vi "Script_Generator.vi"() -> ()   [LabVIEW 2013]
uses:
  Global_Not-Aus.vi
  <vilib>/Utility/file.llb/Read From Spreadsheet File (string).vi
  <vilib>/Utility/file.llb/Write To Spreadsheet File (string).vi
panel:
  out "Abs_pos":string[](array[string])
  out "Array - String":string[][](array[string])
  in  "Main Tab":enum32{"Page 1"}(tab)
  out "Generated Sequence":string[][](array[string])
  in  "Set/Write/Read":enum32{"Position Set", "Write", "Read"}(tab)
  in  "Position Set":T1(tab)
  in  "Generate P1":bool
  in  "Speed (P)":dbl min=0.0 max=20.0
  in  "Generate P2":bool
  in  "Position":T2(ring)
  in  "Proceed W/R":bool
  in  "Generate P3":bool
  in  "Z(P)":string(combo)
  in  "Y(P)":string(combo)
  in  "X(P)":string(combo)
  in  "Z axis":dbl
  in  "Y axis":dbl
  in  "X axis":dbl
  in  "Write_Menu":T3(tab)
  in  "Generate W1":bool
  in  "Speed (W)":dbl min=0.0 max=20.0
  in  "Proceed Inc/Abs":bool
  in  "Current":dbl min=0.0 max=10.0 step=0.1
  in  "Generate W2":bool
  in  "Incre/abs":enum32{"Incremental", "Absolute"}(tab)
  in  "Z_axis(Inc)":string(combo)
  in  "Y_axis(Inc)":string(combo)
  in  "X_axis(Inc)":string(combo)
  in  "Z_axis":dbl
  in  "Y_axis":dbl
  in  "X_axis":dbl
  in  "Incremental":bool
  in  "Strip Length":dbl
  in  "Pole width N":dbl min=0.0 max=10.0 step=0.1
  in  "Pole width S":dbl min=0.0 max=10.0 step=0.1
  in  "Start Pole (N/S)":string(combo)
  in  "Z_axis(Abs)":string(combo)
  in  "Y_axis(Abs)":string(combo)
  in  "X_axis(Abs)":string(combo)
  in  "Start_Pole(N/S)":string(combo)
  in  "Absolute":bool
  in  "Select File":path=path "Y:/01_Projekte/EPN93031_Schreibplatz/8_Konstruktionsunterlagen/8.5_Software/COPY_KOSY Steuerung LabVIEW/1.New_Code_2014_2015/noniuos_scale.txt"
  in  "Generate W4":bool
  in  "File Path_Write":path=path "Y:/01_Projekte/EPN93031_Schreibplatz/8_Konstruktionsunterlagen/8.5_Software/COPY_KOSY Steuerung LabVIEW/1.New_Code_2014_2015/New_Scripts/sample_write.txt"
  in  "Read_Menu":T4(tab)
  in  "Generate R1":bool
  in  "Z(R)":string(combo)
  in  "Y(R)":string(combo)
  in  "X(R)":string(combo)
  in  "Zaxis":dbl min=0.0 max=10.0 step=0.1 format="%#_6f"
  in  "Yaxis":dbl min=0.0 max=10.0 step=0.1 format="%#_2f"
  in  "Xaxis":dbl min=0.0 max=10.0 step=0.1 format="%#_6f"
  out "Count":dbl
  in  "Strip_Length":dbl
  in  "Move&Measure":bool
  in  "Continuous":bool
  in  "Generate R2":bool
  in  "ED32i":bool
  in  "ED33":bool
  in  "KMT":bool
  in  "Generate R4":bool
  in  "File Path_Read":path=path "Y:/01_Projekte/EPN93031_Schreibplatz/8_Konstruktionsunterlagen/8.5_Software/COPY_KOSY Steuerung LabVIEW/1.New_Code_2014_2015/New_Scripts/sample_read.txt"
  in  "Clear Sequence":bool
  in  "Stop Program":bool
  # "SCRIPT GENERATOR  V1.0"
  # "Position Set\n\n1. Speed - Set the speed for the movement to initial \n                   position and press 'OK'.\n2. Batch Position - Select the 'Position' from the dropdown \n                   and press 'OK'.\n3. Movement - Select the number of steps(in mm) for \n                    movement in corresponding axis and also \n                    the direction of travel in the selected axis. \n                    Then press 'OK'."
  # "Speed - Set the speed for the writing process \n                and press 'OK'."
  # "Power - Set the 'Current' from the writing head \n                and press 'OK'."
  # "Incremental Writing Process\n \n1.Set the total 'length' of the strip.\n2.Set the 'Pole width N & S' to be magnetised.\n3.Select the N/S for the initial pole tab. \n3.Set the direction of travel in the selected axis.\n   Then press 'OK'."
  # "Absolute Writing\n\n1. Select the file from 'Select File' for nonious scale.\n2.Select the N/S for the initial pole tab. \n3.Set the direction of travel in the selected axis.\n   Then press 'OK'."
  # "Save Script - Select the file to which the generated \n                         script should be saved and the press 'OK'."
  # "Read\n\n1. Step & Count - 1. Set the total 'length' of the strip.\n                                 2. The 'Count' is automatically generated.\n                                 3. Set the number of steps(in mm) for \n                                     movement in corresponding axis and\n                                     also the direction of travel in the \n                                     selected axis. Then press 'OK'.\n2. Sensors -           Select the 'sensors' to be activated and \n                                 the type of measurement. Then press 'OK'.\n3. Save Script  -    Select the file to which the generated \n                                 script should be saved and the press 'OK'."
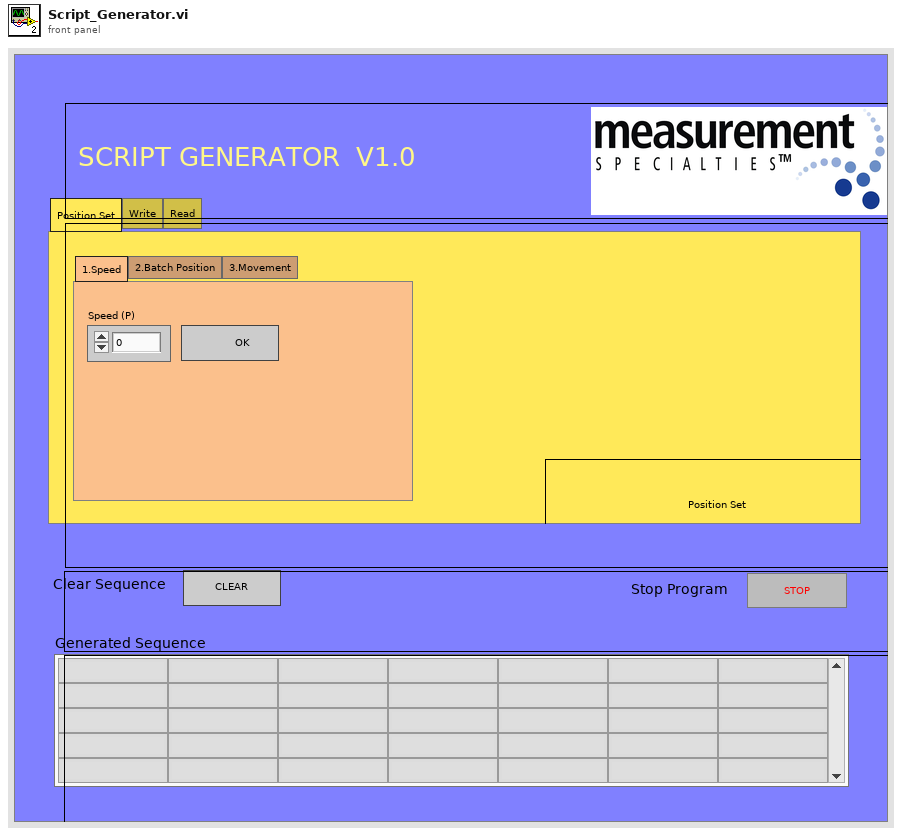
[diagram p1: front panel]
types:
  T1 = enum32{"1.Speed", "2.Batch Position", "3.Movement"}
  T2 = enum16{"Position 1", "Position 2", "Position 3", "Position 4", "Position 5", "Position 6", "Position 7", "Position 8", "Position 9", "Position 10"}
  T3 = enum32{"1.Speed", "2.Power", "3.Movement", "4.Save Script"}
  T4 = enum32{"1.Steps & Count", "2.Sensors", "3.Save Script"}
  T5 = enum16{"1.Speed", "2.Batch Position", "3.Movement"}
  T6 = enum32{"Page Enabled", "Page Disabled", "Page Disabled & Grayed"}
  T7 = enum16{"1.Steps & Count", "2.Sensors", "3.Save Script"}
  T8 = enum16{"1.Speed", "2.Power", "3.Movement", "4.Save Script"}
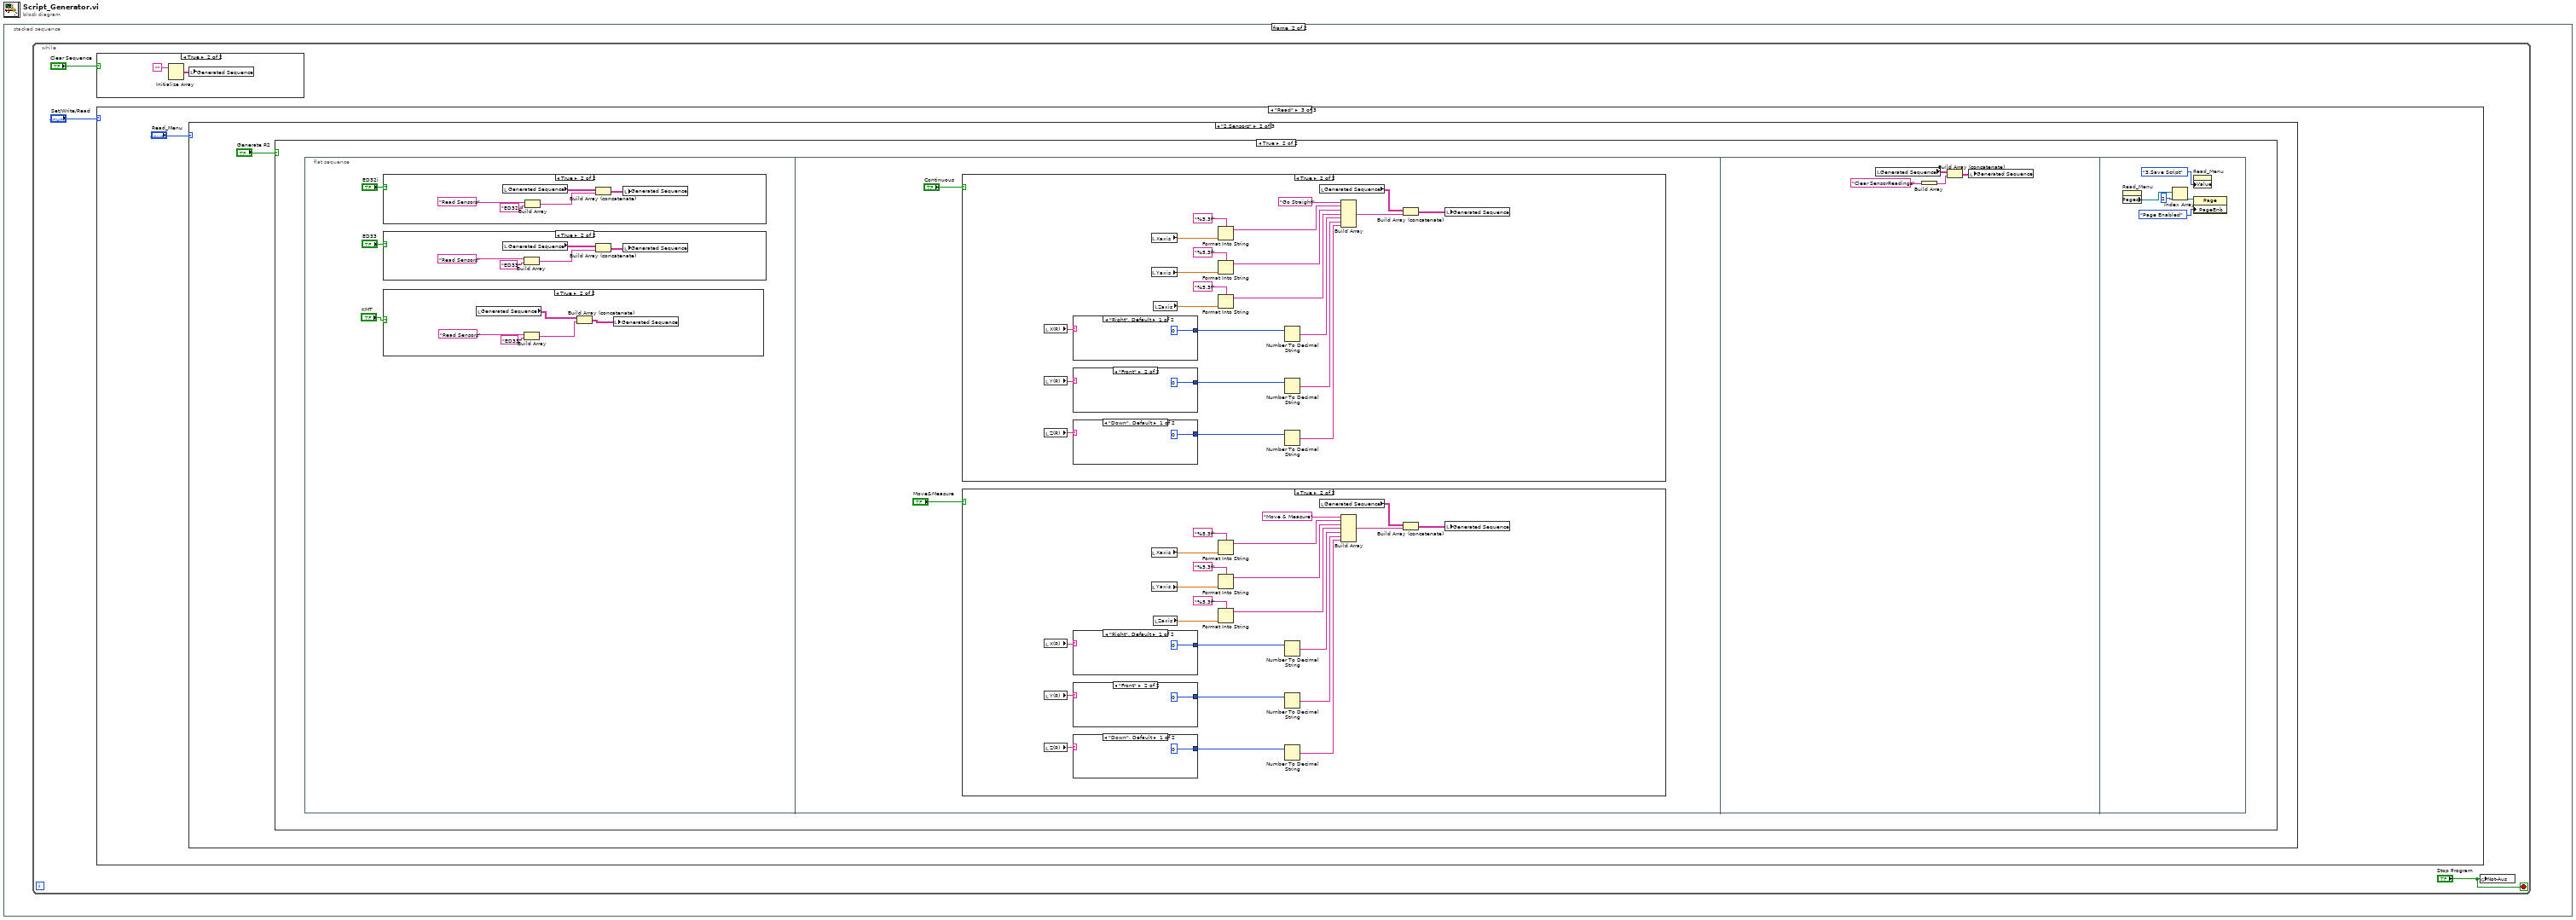
[diagram p0: block diagram]
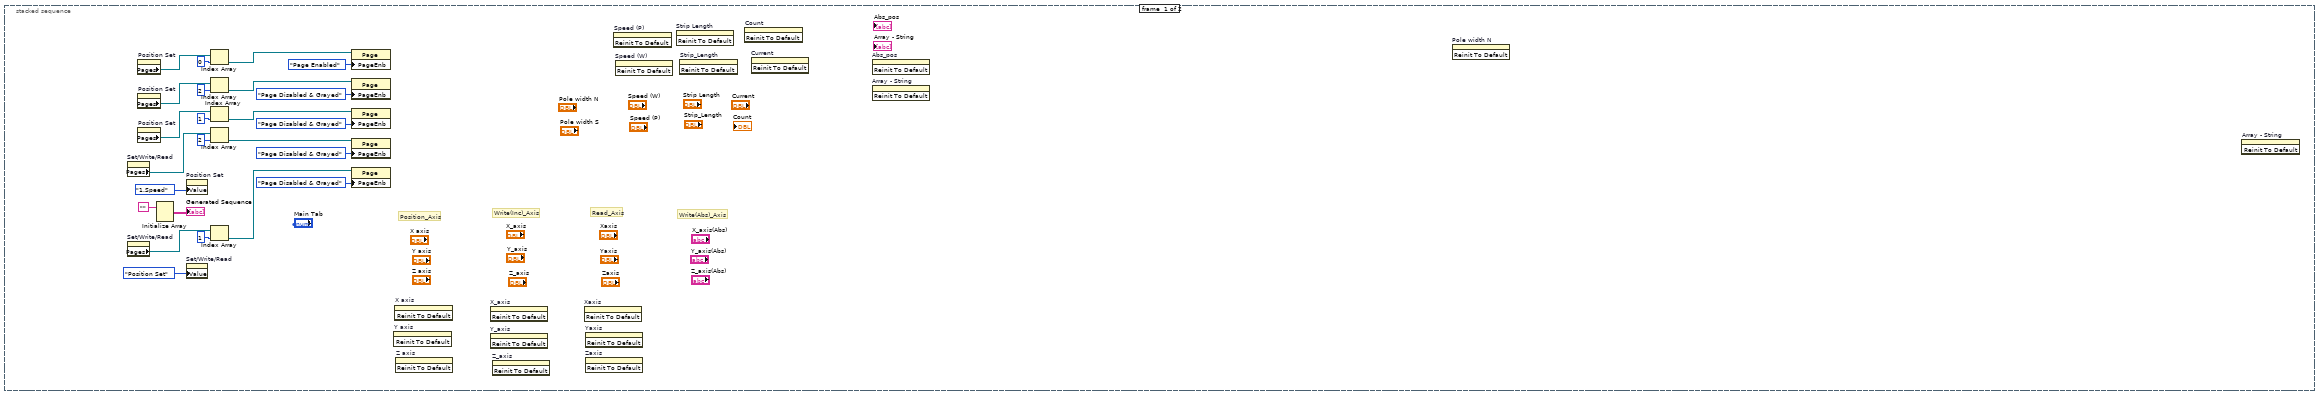
[diagram p2: hidden frame]
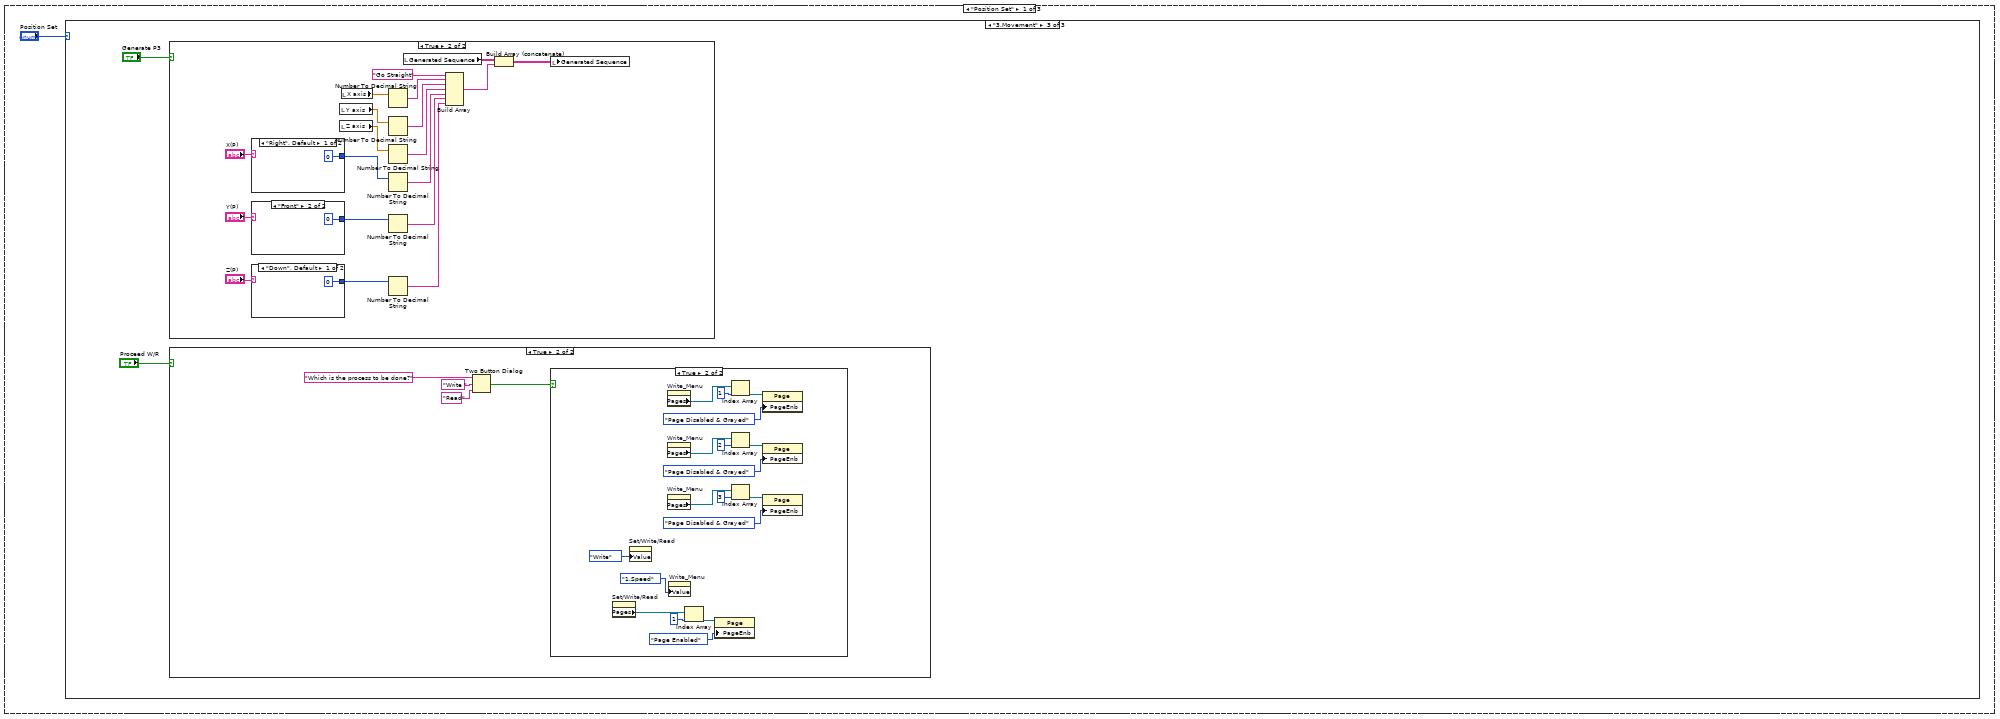
[diagram p4: hidden frame]
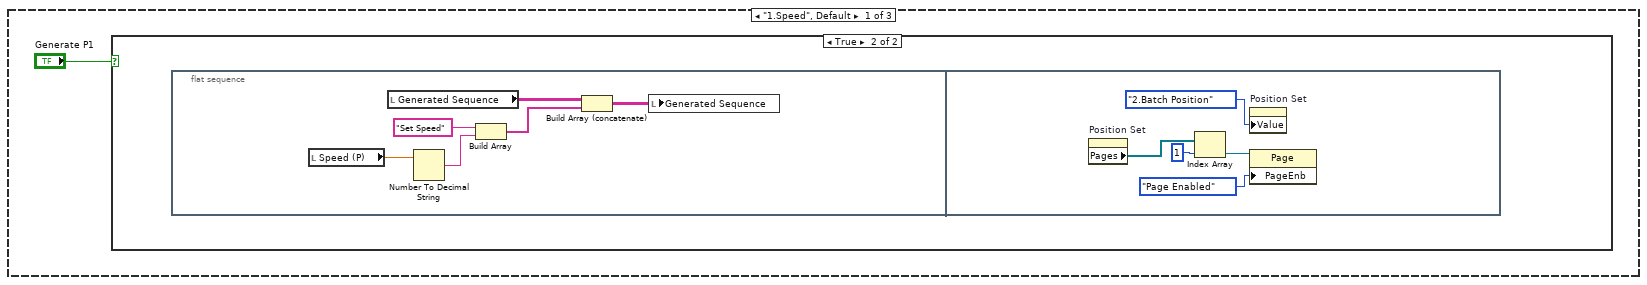
[diagram p5: hidden frame]
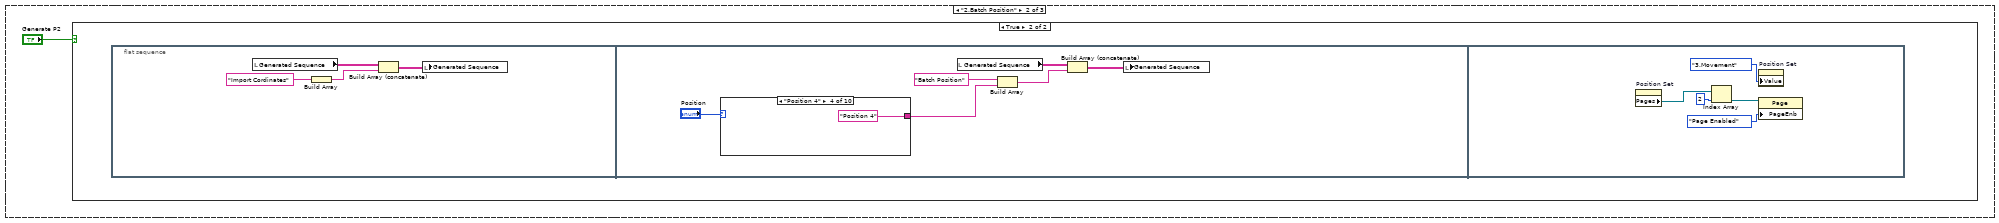
[diagram p7: hidden frame]
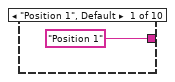
[diagram p9: hidden frame]
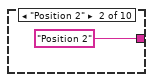
[diagram p10: hidden frame]
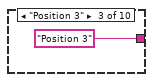
[diagram p11: hidden frame]
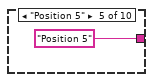
[diagram p12: hidden frame]
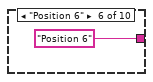
[diagram p13: hidden frame]
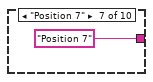
[diagram p14: hidden frame]
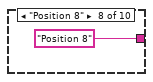
[diagram p15: hidden frame]
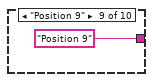
[diagram p16: hidden frame]
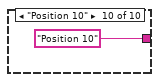
[diagram p17: hidden frame]
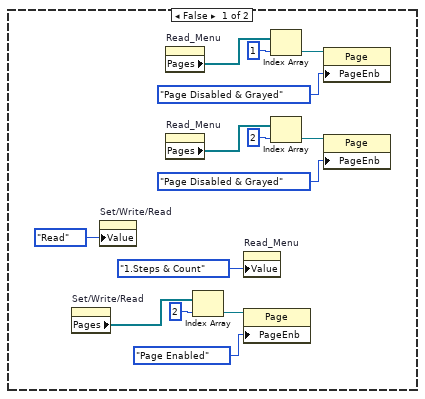
[diagram p19: hidden frame]
diagram:
  n1 = stacked-sequence {
    frame #0 {
      # "Write(Abs)_Axis"
      # "Read_Axis"
      # "Write(Inc)_Axis"
      # "Position_Axis"
      n2 = property on="Set/Write/Read" class="TabCtl (strict)"() -> ("Pages"=w16:refnum<vi>[])  [unwired: 2 in, 2 out]
      n3 = property on="Set/Write/Read" class="TabCtl (strict)"() -> ("Pages"=w15:refnum<vi>[])  [unwired: 2 in, 2 out]
      n4 = property on="Position Set" class="TabCtl (strict)"() -> ("Pages"=w14:refnum<vi>[])  [unwired: 2 in, 2 out]
      n5 = property on="Position Set" class="TabCtl (strict)"() -> ("Pages"=w13:refnum<vi>[])  [unwired: 2 in, 2 out]
      n6 = property on="Position Set" class="TabCtl (strict)"() -> ("Pages"=w3:refnum<vi>[])  [unwired: 2 in, 2 out]
      n7 = Initialize Array("") -> (→"Generated Sequence":string[][])  [unwired: 2 in]
      n8 = property on="Position Set" class="TabCtl (strict)"("Value"=T5."1.Speed") -> ()  [unwired: 2 in, 2 out]
      n9 = property on="Set/Write/Read" class="TabCtl (strict)"("Value"=enum16{"Position Set", "Write", "Read"}."Position Set") -> ()  [unwired: 2 in, 2 out]
      n10 = Index Array(array=w14, index=0) -> (element=w9:refnum<vi>)
      n11 = Index Array(array=w13, index=2) -> (element=w12:refnum<vi>)
      n12 = Index Array(array=w3, index=1) -> (element=w6:refnum<vi>)
      n13 = Index Array(array=w16, index=2) -> (element=w17:refnum<vi>)
      n14 = Index Array(array=w15, index=1) -> (element=w20:refnum<vi>)
      n15 = property class="Page"(reference=w9, "PageEnb"=T6."Page Enabled" ("Page Enabled State")) -> ()  [unwired: 1 in, 2 out]
      n16 = property class="Page"(reference=w12, "PageEnb"=T6."Page Disabled & Grayed" ("Page Enabled State")) -> ()  [unwired: 1 in, 2 out]
      n17 = property class="Page"(reference=w6, "PageEnb"=T6."Page Disabled & Grayed" ("Page Enabled State")) -> ()  [unwired: 1 in, 2 out]
      n18 = property class="Page"(reference=w17, "PageEnb"=T6."Page Disabled & Grayed" ("Page Enabled State")) -> ()  [unwired: 1 in, 2 out]
      n19 = property class="Page"(reference=w20, "PageEnb"=T6."Page Disabled & Grayed" ("Page Enabled State")) -> ()  [unwired: 1 in, 2 out]
      n20 = invoke on="Y axis" class="DigNum (strict)" method="Reinit To Default"() -> ()  [unwired: 3 in, 3 out]
      n21 = invoke on="X axis" class="DigNum (strict)" method="Reinit To Default"() -> ()  [unwired: 3 in, 3 out]
      n22 = invoke on="Z axis" class="DigNum (strict)" method="Reinit To Default"() -> ()  [unwired: 3 in, 3 out]
      n23 = invoke on="X_axis" class="DigNum (strict)" method="Reinit To Default"() -> ()  [unwired: 3 in, 3 out]
      n24 = invoke on="Y_axis" class="DigNum (strict)" method="Reinit To Default"() -> ()  [unwired: 3 in, 3 out]
      n25 = invoke on="Z_axis" class="DigNum (strict)" method="Reinit To Default"() -> ()  [unwired: 3 in, 3 out]
      n26 = invoke on="Xaxis" class="DigNum (strict)" method="Reinit To Default"() -> ()  [unwired: 3 in, 3 out]
      n27 = invoke on="Yaxis" class="DigNum (strict)" method="Reinit To Default"() -> ()  [unwired: 3 in, 3 out]
      n28 = invoke on="Zaxis" class="DigNum (strict)" method="Reinit To Default"() -> ()  [unwired: 3 in, 3 out]
      n29 = invoke on="Speed (P)" class="DigNum (strict)" method="Reinit To Default"() -> ()  [unwired: 3 in, 3 out]
      n30 = invoke on="Speed (W)" class="DigNum (strict)" method="Reinit To Default"() -> ()  [unwired: 3 in, 3 out]
      n31 = invoke on="Strip Length" class="DigNum (strict)" method="Reinit To Default"() -> ()  [unwired: 3 in, 3 out]
      n32 = invoke on="Strip_Length" class="DigNum (strict)" method="Reinit To Default"() -> ()  [unwired: 3 in, 3 out]
      n33 = invoke on="Count" class="DigNum (strict)" method="Reinit To Default"() -> ()  [unwired: 3 in, 3 out]
      n34 = invoke on="Current" class="DigNum (strict)" method="Reinit To Default"() -> ()  [unwired: 3 in, 3 out]
      n35 = invoke on="Abs_pos" class="Arr (strict)" method="Reinit To Default"() -> ()  [unwired: 3 in, 3 out]
      n36 = invoke on="Array - String" class="Arr (strict)" method="Reinit To Default"() -> ()  [unwired: 3 in, 3 out]
      n37 = invoke on="Pole width N" class="DigNum (strict)" method="Reinit To Default"() -> ()  [unwired: 3 in, 3 out]
      n38 = invoke on="Array - String" class="Arr (strict)" method="Reinit To Default"() -> ()  [unwired: 3 in, 3 out]
    }
    frame #1 {
      n39 = while {
        stop <- "Stop Program" stop-if-true
        n40 = case shown="True" "Clear Sequence" {
          frame False {
          }
          frame True {
            n41 = Initialize Array("") -> (w29:string[][])  [unwired: 2 in]
            n42 = local write "Generated Sequence"(w29) -> ()
          }
        }
        n43 = case shown="\"Read\"" "Set/Write/Read" {
          frame "Position Set" {
            n44 = case shown="\"3.Movement\"" "Position Set" {
              frame "1.Speed", Default {
                n45 = case shown="True" "Generate P1" {
                  frame False {
                  }
                  frame True {
                    n46 = flat-sequence {
                      frame #0 {
                        n47 = local read "Speed (P)"() -> (w37:dbl)
                        n48 = local read "Generated Sequence"() -> (w35:string[][])
                        n49 = Number To Decimal String(number=w37) -> (decimal integer string=w32:string)  [unwired: 1 in]
                        n50 = Build Array("Set Speed", w32) -> (w34:string[])
                        n51 = Build Array (concatenate)(w35, w34) -> (w36:string[][])
                        n52 = local write "Generated Sequence"(w36) -> ()
                      }
                      frame #1 {
                        n53 = property on="Position Set" class="TabCtl (strict)"() -> ("Pages"=w39:refnum<vi>[])  [unwired: 2 in, 2 out]
                        n54 = Index Array(array=w39, index=1) -> (element=w42:refnum<vi>)
                        n55 = property on="Position Set" class="TabCtl (strict)"("Value"=T5."2.Batch Position") -> ()  [unwired: 2 in, 2 out]
                        n56 = property class="Page"(reference=w42, "PageEnb"=T6."Page Enabled" ("Page Enabled State")) -> ()  [unwired: 1 in, 2 out]
                      }
                    }
                  }
                }
              }
              frame "2.Batch Position" {
                n57 = case shown="True" "Generate P2" {
                  frame False {
                  }
                  frame True {
                    n58 = flat-sequence {
                      frame #0 {
                        n59 = local read "Generated Sequence"() -> (w47:string[][])
                        n60 = Build Array("Import Cordinates") -> (w46:string[])
                        n61 = Build Array (concatenate)(w47, w46) -> (w44:string[][])
                        n62 = local write "Generated Sequence"(w44) -> ()
                      }
                      frame #1 {
                        n63 = case shown="\"Position 4\"" "Position" {
                          tunnel: ["Position 1" "Position 2" "Position 3" "Position 4" "Position 5" "Position 6" "Position 7" "Position 8" "Position 9" "Position 10"] -> w52
                          frame "Position 1", Default {
                          }
                          frame "Position 2" {
                          }
                          frame "Position 3" {
                          }
                          frame "Position 4" {
                          }
                          frame "Position 5" {
                          }
                          frame "Position 6" {
                          }
                          frame "Position 7" {
                          }
                          frame "Position 8" {
                          }
                          frame "Position 9" {
                          }
                          frame "Position 10" {
                          }
                        }
                        n64 = local read "Generated Sequence"() -> (w50:string[][])
                        n65 = Build Array("Batch Position", w52) -> (w51:string[])
                        n66 = Build Array (concatenate)(w50, w51) -> (w49:string[][])
                        n67 = local write "Generated Sequence"(w49) -> ()
                      }
                      frame #2 {
                        n68 = property on="Position Set" class="TabCtl (strict)"() -> ("Pages"=w65:refnum<vi>[])  [unwired: 2 in, 2 out]
                        n69 = Index Array(array=w65, index=2) -> (element=w68:refnum<vi>)
                        n70 = property on="Position Set" class="TabCtl (strict)"("Value"=T5."3.Movement") -> ()  [unwired: 2 in, 2 out]
                        n71 = property class="Page"(reference=w68, "PageEnb"=T6."Page Enabled" ("Page Enabled State")) -> ()  [unwired: 1 in, 2 out]
                      }
                    }
                  }
                }
              }
              frame "3.Movement" {
                n72 = case shown="True" "Generate P3" {
                  frame False {
                  }
                  frame True {
                    n73 = case shown="\"Right\", Default" "X(P)" {
                      tunnel: [0 1] -> w110
                      frame "Right", Default {
                      }
                      frame "Left" {
                      }
                    }
                    n74 = case shown="\"Front\"" "Y(P)" {
                      tunnel: [1 0] -> w111
                      frame "Back", Default {
                      }
                      frame "Front" {
                      }
                    }
                    n75 = case shown="\"Down\", Default" "Z(P)" {
                      tunnel: [0 1] -> w112
                      frame "Down", Default {
                      }
                      frame "Up" {
                      }
                    }
                    n76 = local read "Y axis"() -> (w124:dbl)
                    n77 = local read "Z axis"() -> (w125:dbl)
                    n78 = local read "X axis"() -> (w123:dbl)
                    n79 = Number To Decimal String(number=w123) -> (decimal integer string=w114:string)  [unwired: 1 in]
                    n80 = Number To Decimal String(number=w124) -> (decimal integer string=w115:string)  [unwired: 1 in]
                    n81 = Number To Decimal String(number=w125) -> (decimal integer string=w116:string)  [unwired: 1 in]
                    n82 = Number To Decimal String(number=w110) -> (decimal integer string=w117:string)  [unwired: 1 in]
                    n83 = Number To Decimal String(number=w111) -> (decimal integer string=w118:string)  [unwired: 1 in]
                    n84 = Number To Decimal String(number=w112) -> (decimal integer string=w119:string)  [unwired: 1 in]
                    n85 = local read "Generated Sequence"() -> (w121:string[][])
                    n86 = Build Array("Go Straight", w114, w115, w116, w117, w118, w119) -> (w120:string[])
                    n87 = Build Array (concatenate)(w121, w120) -> (w122:string[][])
                    n88 = local write "Generated Sequence"(w122) -> ()
                  }
                }
                n89 = case shown="True" "Proceed W/R" {
                  frame False {
                  }
                  frame True {
                    n90 = Two Button Dialog(message="Which is the process to be done?", 1:"Read" ("F button name (\"Cancel\")"), 2:"Write " ("T button name (\"OK\")")) -> (T button?=w74:bool)
                    n91 = case shown="True" w74 {
                      frame False {
                        n92 = property on="Set/Write/Read" class="TabCtl (strict)"() -> ("Pages"=w85:refnum<vi>[])  [unwired: 2 in, 2 out]
                        n93 = property on="Set/Write/Read" class="TabCtl (strict)"("Value"=enum16{"Position Set", "Write", "Read"}."Read") -> ()  [unwired: 2 in, 2 out]
                        n94 = property on="Read_Menu" class="TabCtl (strict)"() -> ("Pages"=w77:refnum<vi>[])  [unwired: 2 in, 2 out]
                        n95 = property on="Read_Menu" class="TabCtl (strict)"() -> ("Pages"=w78:refnum<vi>[])  [unwired: 2 in, 2 out]
                        n96 = Index Array(array=w85, index=2) -> (element=w86:refnum<vi>)
                        n97 = property on="Read_Menu" class="TabCtl (strict)"("Value"=T7."1.Steps & Count") -> ()  [unwired: 2 in, 2 out]
                        n98 = property class="Page"(reference=w86, "PageEnb"=T6."Page Enabled" ("Page Enabled State")) -> ()  [unwired: 1 in, 2 out]
                        n99 = Index Array(array=w77, index=1) -> (element=w79:refnum<vi>)
                        n100 = Index Array(array=w78, index=2) -> (element=w82:refnum<vi>)
                        n101 = property class="Page"(reference=w79, "PageEnb"=T6."Page Disabled & Grayed" ("Page Enabled State")) -> ()  [unwired: 1 in, 2 out]
                        n102 = property class="Page"(reference=w82, "PageEnb"=T6."Page Disabled & Grayed" ("Page Enabled State")) -> ()  [unwired: 1 in, 2 out]
                      }
                      frame True {
                        n103 = property on="Set/Write/Read" class="TabCtl (strict)"() -> ("Pages"=w103:refnum<vi>[])  [unwired: 2 in, 2 out]
                        n104 = property on="Set/Write/Read" class="TabCtl (strict)"("Value"=enum16{"Position Set", "Write", "Read"}."Write") -> ()  [unwired: 2 in, 2 out]
                        n105 = property on="Write_Menu" class="TabCtl (strict)"() -> ("Pages"=w96:refnum<vi>[])  [unwired: 2 in, 2 out]
                        n106 = property on="Write_Menu" class="TabCtl (strict)"() -> ("Pages"=w95:refnum<vi>[])  [unwired: 2 in, 2 out]
                        n107 = property on="Write_Menu" class="TabCtl (strict)"() -> ("Pages"=w91:refnum<vi>[])  [unwired: 2 in, 2 out]
                        n108 = property on="Write_Menu" class="TabCtl (strict)"("Value"=T8."1.Speed") -> ()  [unwired: 2 in, 2 out]
                        n109 = Index Array(array=w103, index=1) -> (element=w104:refnum<vi>)
                        n110 = property class="Page"(reference=w104, "PageEnb"=T6."Page Enabled" ("Page Enabled State")) -> ()  [unwired: 1 in, 2 out]
                        n111 = Index Array(array=w96, index=1) -> (element=w100:refnum<vi>)
                        n112 = Index Array(array=w95, index=2) -> (element=w97:refnum<vi>)
                        n113 = Index Array(array=w91, index=3) -> (element=w92:refnum<vi>)
                        n114 = property class="Page"(reference=w100, "PageEnb"=T6."Page Disabled & Grayed" ("Page Enabled State")) -> ()  [unwired: 1 in, 2 out]
                        n115 = property class="Page"(reference=w97, "PageEnb"=T6."Page Disabled & Grayed" ("Page Enabled State")) -> ()  [unwired: 1 in, 2 out]
                        n116 = property class="Page"(reference=w92, "PageEnb"=T6."Page Disabled & Grayed" ("Page Enabled State")) -> ()  [unwired: 1 in, 2 out]
                      }
                    }
                  }
                }
              }
            }
          }
          frame "Write", Default {
            n117 = case shown="\"3.Movement\"" "Write_Menu" {
              frame "1.Speed", Default {
                n118 = case shown="True" "Generate W1" {
                  frame False {
                  }
                  frame True {
                    n119 = flat-sequence {
                      frame #0 {
                        n120 = local read "Speed (W)"() -> (w139:dbl)
                        n121 = local read "Generated Sequence"() -> (w137:string[][])
                        n122 = Number To Decimal String(number=w139) -> (decimal integer string=w134:string)  [unwired: 1 in]
                        n123 = Build Array("Set Speed", w134) -> (w136:string[])
                        n124 = Build Array (concatenate)(w137, w136) -> (w138:string[][])
                        n125 = local write "Generated Sequence"(w138) -> ()
                      }
                      frame #1 {
                        n126 = property on="Write_Menu" class="TabCtl (strict)"() -> ("Pages"=w141:refnum<vi>[])  [unwired: 2 in, 2 out]
                        n127 = property on="Write_Menu" class="TabCtl (strict)"("Value"=T8."2.Power") -> ()  [unwired: 2 in, 2 out]
                        n128 = Index Array(array=w141, index=1) -> (element=w142:refnum<vi>)
                        n129 = property class="Page"(reference=w142, "PageEnb"=T6."Page Enabled" ("Page Enabled State")) -> ()  [unwired: 1 in, 2 out]
                      }
                    }
                  }
                }
              }
              frame "2.Power" {
                n130 = case shown="True" "Generate W2" {
                  frame False {
                  }
                  frame True {
                    n131 = flat-sequence {
                      frame #0 {
                        n132 = local read "Current"() -> (w175:dbl)
                        n133 = Number To Decimal String(number=w175) -> (decimal integer string=w174:string)  [unwired: 1 in]
                        n134 = Concatenate Strings("GPC", "  ", w174) -> (w178:string)
                        n135 = local read "Generated Sequence"() -> (w181:string[][])
                        n136 = Build Array("Set Powersupply", w178) -> (w180:string[])
                        n137 = Build Array (concatenate)(w181, w180) -> (w182:string[][])
                        n138 = local write "Generated Sequence"(w182) -> ()
                      }
                    }
                  }
                }
                n139 = case shown="True" "Proceed Inc/Abs" {
                  frame False {
                  }
                  frame True {
                    n140 = property on="Write_Menu" class="TabCtl (strict)"() -> ("Pages"=w150:refnum<vi>[])  [unwired: 2 in, 2 out]
                    n141 = Index Array(array=w150, index=2) -> (element=w149:refnum<vi>)
                    n142 = property class="Page"(reference=w149, "PageEnb"=T6."Page Enabled" ("Page Enabled State")) -> ()  [unwired: 1 in, 2 out]
                    n143 = Two Button Dialog(message="Writing method ?", 1:"Absolute" ("F button name (\"Cancel\")"), 2:"Incremental" ("T button name (\"OK\")")) -> (T button?=w154:bool)
                    n144 = case shown="False" w154 {
                      frame False {
                        (unwired) 0 ("index")
                        n145 = property on="Incre/abs" class="TabCtl (strict)"() -> ("Pages"=w161:refnum<vi>[])  [unwired: 2 in, 2 out]
                        n146 = property on="Incre/abs" class="TabCtl (strict)"("Value"=enum16{"Incremental", "Absolute"}."Absolute") -> ()  [unwired: 2 in, 2 out]
                        n147 = property on="Incre/abs" class="TabCtl (strict)"() -> ("Pages"=w163:refnum<vi>[])  [unwired: 2 in, 2 out]
                        n148 = Index Array(array=w161, index=1) -> (element=w160:refnum<vi>)
                        n149 = property on="Write_Menu" class="TabCtl (strict)"("Value"=T8."3.Movement") -> ()  [unwired: 2 in, 2 out]
                        n150 = property class="Page"(reference=w160, "PageEnb"=T6."Page Enabled" ("Page Enabled State")) -> ()  [unwired: 1 in, 2 out]
                        n151 = Index Array(array=w163) -> (element=w162:refnum<vi>)  [unwired: 1 in]
                        n152 = property class="Page"(reference=w162, "PageEnb"=T6."Page Disabled & Grayed" ("Page Enabled State")) -> ()  [unwired: 1 in, 2 out]
                      }
                      frame True {
                        n153 = property on="Incre/abs" class="TabCtl (strict)"() -> ("Pages"=w172:refnum<vi>[])  [unwired: 2 in, 2 out]
                        n154 = property on="Incre/abs" class="TabCtl (strict)"("Value"=enum16{"Incremental", "Absolute"}."Incremental") -> ()  [unwired: 2 in, 2 out]
                        n155 = property on="Incre/abs" class="TabCtl (strict)"() -> ("Pages"=w165:refnum<vi>[])  [unwired: 2 in, 2 out]
                        n156 = Index Array(array=w172, index=0) -> (element=w171:refnum<vi>)
                        n157 = property class="Page"(reference=w171, "PageEnb"=T6."Page Enabled" ("Page Enabled State")) -> ()  [unwired: 1 in, 2 out]
                        n158 = property on="Write_Menu" class="TabCtl (strict)"("Value"=T8."3.Movement") -> ()  [unwired: 2 in, 2 out]
                        n159 = Index Array(array=w165, index=1) -> (element=w168:refnum<vi>)
                        n160 = property class="Page"(reference=w168, "PageEnb"=T6."Page Disabled & Grayed" ("Page Enabled State")) -> ()  [unwired: 1 in, 2 out]
                      }
                    }
                  }
                }
              }
              frame "3.Movement" {
                n161 = case shown="\"Absolute\"" "Incre/abs" {
                  frame "Absolute" {
                    n162 = case shown="True" "Absolute" {
                      frame False {
                      }
                      frame True {
                        n163 = call-poly <vilib>:"Read From Spreadsheet File.vi"("file path (dialog if empty)"="Select File") -> ("all rows"=w185:string[][])  [unwired: 6 in, 4 out]
                        n164 = local read "Array - String"() -> (w188:string[][])
                        n165 = local write "Array - String"(w185) -> ()
                        n166 = case shown="\"South\"" "Start_Pole(N/S)" {
                          frame "South" {
                            n167 = flat-sequence {
                              frame #0 {
                                n168 = while {
                                stop <- w193 stop-if-true
                                n169 = flat-sequence {
                                frame #0 {
                                n170 = stacked-sequence {
                                frame #0 {
                                n171 = local read "Generated Sequence"() -> (w195:string[][])
                                n172 = Build Array("Write  Pole", "N", "0", "0", "0", "0") -> (w196:string[])
                                n173 = Build Array (concatenate)(w195, w196) -> (w194:string[][])
                                n174 = local write "Generated Sequence"(w194) -> ()
                                }
                                frame #1 {
                                n175 = local read "X_axis(Abs)"() -> (w205:string)
                                n176 = local read "Y_axis(Abs)"() -> (w204:string)
                                n177 = local read "Z_axis(Abs)"() -> (w203:string)
                                n178 = local read "Array - String"() -> (w223:string[][])
                                n179 = case shown="\"Right\", Default" w205 {
                                tunnel: [0 1] -> w212
                                frame "Right", Default {
                                }
                                frame "Left" {
                                }
                                }
                                n180 = case shown="\"Back\", Default" w204 {
                                tunnel: [1 0] -> w213
                                frame "Back", Default {
                                }
                                frame "Front" {
                                }
                                }
                                n181 = case shown="\"Down\", Default" w203 {
                                tunnel: [0 1] -> w214
                                frame "Down", Default {
                                }
                                frame "Up" {
                                }
                                }
                                n182 = Delete From Array(array=w223, index (row)=0) -> (deleted portion=w206:string[], array with subset deleted=w222:string[][])  [unwired: 2 in]
                                n183 = local write "Array - String"(w222) -> ()
                                n184 = local write "Abs_pos"(w206) -> ()
                                n185 = local read "Abs_pos"() -> (w209:string[])
                                n186 = Number To Decimal String(number=w212) -> (decimal integer string=w218:string)  [unwired: 1 in]
                                n187 = Number To Decimal String(number=w213) -> (decimal integer string=w219:string)  [unwired: 1 in]
                                n188 = Number To Decimal String(number=w214) -> (decimal integer string=w220:string)  [unwired: 1 in]
                                n189 = Number To Decimal String(number=0) -> (decimal integer string=w216:string)  [unwired: 1 in]
                                n190 = Number To Decimal String(number=0) -> (decimal integer string=w217:string)  [unwired: 1 in]
                                n191 = local read "Generated Sequence"() -> (w208:string[][])
                                n192 = Build Array (concatenate)("Go Straight", w216, w209, w217, w218, w219, w220) -> (w221:string[])
                                n193 = Build Array (concatenate)(w208, w221) -> (w207:string[][])
                                n194 = local write "Generated Sequence"(w207) -> ()
                                }
                                }
                                }
                                frame #1 {
                                n195 = stacked-sequence {
                                frame #0 {
                                n196 = Build Array("Write  Pole", "P", "0", "0", "0", "0") -> (w233:string[])
                                n197 = local read "Generated Sequence"() -> (w232:string[][])
                                n198 = Build Array (concatenate)(w232, w233) -> (w231:string[][])
                                n199 = local write "Generated Sequence"(w231) -> ()
                                }
                                frame #1 {
                                n200 = local read "X_axis(Abs)"() -> (w242:string)
                                n201 = local read "Y_axis(Abs)"() -> (w241:string)
                                n202 = local read "Z_axis(Abs)"() -> (w240:string)
                                n203 = case shown="\"Right\", Default" w242 {
                                tunnel: [0 1] -> w252
                                frame "Right", Default {
                                }
                                frame "Left" {
                                }
                                }
                                n204 = case shown="\"Back\", Default" w241 {
                                tunnel: [1 0] -> w253
                                frame "Back", Default {
                                }
                                frame "Front" {
                                }
                                }
                                n205 = case shown="\"Down\", Default" w240 {
                                tunnel: [0 1] -> w254
                                frame "Down", Default {
                                }
                                frame "Up" {
                                }
                                }
                                n206 = local read "Array - String"() -> (w247:string[][])
                                n207 = Delete From Array(array=w247, index (row)=0) -> (deleted portion=w245:string[], array with subset deleted=w246:string[][])  [unwired: 2 in]
                                n208 = local write "Array - String"(w246) -> ()
                                n209 = local write "Abs_pos"(w245) -> ()
                                n210 = local read "Abs_pos"() -> (w249:string[])
                                n211 = Number To Decimal String(number=w252) -> (decimal integer string=w258:string)  [unwired: 1 in]
                                n212 = Number To Decimal String(number=w253) -> (decimal integer string=w259:string)  [unwired: 1 in]
                                n213 = Number To Decimal String(number=w254) -> (decimal integer string=w260:string)  [unwired: 1 in]
                                n214 = local read "Generated Sequence"() -> (w244:string[][])
                                n215 = Number To Decimal String(number=0) -> (decimal integer string=w256:string)  [unwired: 1 in]
                                n216 = Number To Decimal String(number=0) -> (decimal integer string=w257:string)  [unwired: 1 in]
                                n217 = Build Array (concatenate)("Go Straight", w256, w249, w257, w258, w259, w260) -> (w261:string[])
                                n218 = Build Array (concatenate)(w244, w261) -> (w243:string[][])
                                n219 = local write "Generated Sequence"(w243) -> ()
                                }
                                }
                                }
                                }
                                n220 = local read "Abs_pos"() -> (w192:string[])
                                n221 = Empty Array?(array=w192) -> (empty?=w193:bool)
                                }
                              }
                              frame #1 {
                                n222 = property on="Write_Menu" class="TabCtl (strict)"() -> ("Pages"=w269:refnum<vi>[])  [unwired: 2 in, 2 out]
                                n223 = Index Array(array=w269, index=3) -> (element=w270:refnum<vi>)
                                n224 = property on="Write_Menu" class="TabCtl (strict)"("Value"=T8."4.Save Script") -> ()  [unwired: 2 in, 2 out]
                                n225 = property class="Page"(reference=w270, "PageEnb"=T6."Page Enabled" ("Page Enabled State")) -> ()  [unwired: 1 in, 2 out]
                              }
                            }
                          }
                          frame "North", Default {
                            n226 = flat-sequence {
                              frame #0 {
                                n227 = while {
                                stop <- w274 stop-if-true
                                n228 = flat-sequence {
                                frame #0 {
                                n229 = stacked-sequence {
                                frame #0 {
                                n230 = local read "Abs_pos"() -> (w275:string[])
                                n231 = Empty Array?(array=w275) -> (empty?=w276:bool)
                                n232 = case shown="False" w276 {
                                frame False {
                                n233 = Build Array("Write  Pole", "P", "0", "0", "0", "0") -> (w283:string[])
                                n234 = local read "Generated Sequence"() -> (w284:string[][])
                                n235 = Build Array (concatenate)(w284, w283) -> (w285:string[][])
                                n236 = local write "Generated Sequence"(w285) -> ()
                                }
                                frame True {
                                }
                                }
                                }
                                frame #1 {
                                n237 = local read "X_axis(Abs)"() -> (w290:string)
                                n238 = local read "Y_axis(Abs)"() -> (w289:string)
                                n239 = local read "Z_axis(Abs)"() -> (w288:string)
                                n240 = local read "Array - String"() -> (w293:string[][])
                                n241 = case shown="\"Right\", Default" w290 {
                                tunnel: [0 1] -> w298
                                frame "Right", Default {
                                }
                                frame "Left" {
                                }
                                }
                                n242 = case shown="\"Back\", Default" w289 {
                                tunnel: [1 0] -> w299
                                frame "Back", Default {
                                }
                                frame "Front" {
                                }
                                }
                                n243 = case shown="\"Down\", Default" w288 {
                                tunnel: [0 1] -> w300
                                frame "Down", Default {
                                }
                                frame "Up" {
                                }
                                }
                                n244 = Delete From Array(array=w293, index (row)=0) -> (deleted portion=w291:string[], array with subset deleted=w292:string[][])  [unwired: 2 in]
                                n245 = local write "Array - String"(w292) -> ()
                                n246 = local write "Abs_pos"(w291) -> ()
                                n247 = local read "Abs_pos"() -> (w295:string[])
                                n248 = Number To Decimal String(number=w298) -> (decimal integer string=w304:string)  [unwired: 1 in]
                                n249 = Number To Decimal String(number=w299) -> (decimal integer string=w305:string)  [unwired: 1 in]
                                n250 = Number To Decimal String(number=w300) -> (decimal integer string=w306:string)  [unwired: 1 in]
                                n251 = Number To Decimal String(number=0) -> (decimal integer string=w302:string)  [unwired: 1 in]
                                n252 = Number To Decimal String(number=0) -> (decimal integer string=w303:string)  [unwired: 1 in]
                                n253 = local read "Generated Sequence"() -> (w286:string[][])
                                n254 = Build Array (concatenate)("Go Straight", w302, w295, w303, w304, w305, w306) -> (w307:string[])
                                n255 = Build Array (concatenate)(w286, w307) -> (w287:string[][])
                                n256 = local write "Generated Sequence"(w287) -> ()
                                }
                                }
                                }
                                frame #1 {
                                n257 = stacked-sequence {
                                frame #0 {
                                n258 = local read "Abs_pos"() -> (w314:string[])
                                n259 = Empty Array?(array=w314) -> (empty?=w315:bool)
                                n260 = case shown="False" w315 {
                                frame False {
                                n261 = local read "Generated Sequence"() -> (w324:string[][])
                                n262 = Build Array("Write  Pole", "N", "0", "0", "0", "0") -> (w322:string[])
                                n263 = Build Array (concatenate)(w324, w322) -> (w323:string[][])
                                n264 = local write "Generated Sequence"(w323) -> ()
                                }
                                frame True {
                                }
                                }
                                }
                                frame #1 {
                                n265 = local read "X_axis(Abs)"() -> (w329:string)
                                n266 = local read "Y_axis(Abs)"() -> (w328:string)
                                n267 = local read "Z_axis(Abs)"() -> (w327:string)
                                n268 = case shown="\"Right\", Default" w329 {
                                tunnel: [0 1] -> w337
                                frame "Right", Default {
                                }
                                frame "Left" {
                                }
                                }
                                n269 = case shown="\"Back\", Default" w328 {
                                tunnel: [1 0] -> w338
                                frame "Back", Default {
                                }
                                frame "Front" {
                                }
                                }
                                n270 = case shown="\"Down\", Default" w327 {
                                tunnel: [0 1] -> w339
                                frame "Down", Default {
                                }
                                frame "Up" {
                                }
                                }
                                n271 = local read "Array - String"() -> (w330:string[][])
                                n272 = Delete From Array(array=w330, index (row)=0) -> (deleted portion=w331:string[], array with subset deleted=w332:string[][])  [unwired: 2 in]
                                n273 = local write "Array - String"(w332) -> ()
                                n274 = local write "Abs_pos"(w331) -> ()
                                n275 = local read "Abs_pos"() -> (w334:string[])
                                n276 = Number To Decimal String(number=w337) -> (decimal integer string=w343:string)  [unwired: 1 in]
                                n277 = Number To Decimal String(number=w338) -> (decimal integer string=w344:string)  [unwired: 1 in]
                                n278 = Number To Decimal String(number=w339) -> (decimal integer string=w345:string)  [unwired: 1 in]
                                n279 = local read "Generated Sequence"() -> (w326:string[][])
                                n280 = Number To Decimal String(number=0) -> (decimal integer string=w341:string)  [unwired: 1 in]
                                n281 = Number To Decimal String(number=0) -> (decimal integer string=w342:string)  [unwired: 1 in]
                                n282 = Build Array (concatenate)("Go Straight", w341, w334, w342, w343, w344, w345) -> (w346:string[])
                                n283 = Build Array (concatenate)(w326, w346) -> (w325:string[][])
                                n284 = local write "Generated Sequence"(w325) -> ()
                                }
                                }
                                }
                                }
                                n285 = local read "Abs_pos"() -> (w273:string[])
                                n286 = Empty Array?(array=w273) -> (empty?=w274:bool)
                                }
                              }
                              frame #1 {
                                n287 = property on="Write_Menu" class="TabCtl (strict)"() -> ("Pages"=w353:refnum<vi>[])  [unwired: 2 in, 2 out]
                                n288 = Index Array(array=w353, index=3) -> (element=w354:refnum<vi>)
                                n289 = property on="Write_Menu" class="TabCtl (strict)"("Value"=T8."4.Save Script") -> ()  [unwired: 2 in, 2 out]
                                n290 = property class="Page"(reference=w354, "PageEnb"=T6."Page Enabled" ("Page Enabled State")) -> ()  [unwired: 1 in, 2 out]
                              }
                            }
                          }
                        }
                        n291 = Delete From Array(array=w188, index (row)=0) -> (deleted portion=w186:string[], array with subset deleted=w187:string[][])  [unwired: 2 in]
                        n292 = local write "Array - String"(w187) -> ()
                        n293 = local write "Abs_pos"(w186) -> ()
                      }
                    }
                  }
                  frame "Incremental", Default {
                    n294 = case shown="True" "Incremental" {
                      frame False {
                      }
                      frame True {
                        n295 = case shown="\"South\"" "Start Pole (N/S)" {
                          frame "South" {
                            n296 = flat-sequence {
                              frame #0 {
                                n297 = local read "Pole width N"() -> (w362:dbl)
                                n298 = local read "Pole width S"() -> (w361:dbl)
                                n299 = local read "Strip Length"() -> (w364:dbl)
                                n300 = Add(x=w362, y=w361) -> (x+y=w360:dbl)
                                n301 = Divide(x=w364, y=w360) -> (x/y=w363:dbl)
                                n302 = for {
                                N: w363 -> [_]
                                n303 = flat-sequence {
                                frame #0 {
                                n304 = stacked-sequence {
                                frame #0 {
                                n305 = Build Array("Write  Pole", "N", "0", "0", "0", "0") -> (w366:string[])
                                n306 = local read "Generated Sequence"() -> (w367:string[][])
                                n307 = Build Array (concatenate)(w367, w366) -> (w365:string[][])
                                n308 = local write "Generated Sequence"(w365) -> ()
                                }
                                frame #1 {
                                n309 = local read "X_axis(Inc)"() -> (w376:string)
                                n310 = local read "Y_axis(Inc)"() -> (w377:string)
                                n311 = local read "Z_axis(Inc)"() -> (w378:string)
                                n312 = case shown="\"Right\", Default" w376 {
                                tunnel: [0 1] -> w380
                                frame "Right", Default {
                                }
                                frame "Left" {
                                }
                                }
                                n313 = case shown="\"Back\", Default" w377 {
                                tunnel: [1 0] -> w381
                                frame "Back", Default {
                                }
                                frame "Front" {
                                }
                                }
                                n314 = case shown="\"Down\", Default" w378 {
                                tunnel: [0 1] -> w382
                                frame "Down", Default {
                                }
                                frame "Up" {
                                }
                                }
                                n315 = local read "Pole width S"() -> (w379:dbl)
                                n316 = Number To Decimal String(number=w379) -> (decimal integer string=w385:string)  [unwired: 1 in]
                                n317 = Number To Decimal String(number=w380) -> (decimal integer string=w387:string)  [unwired: 1 in]
                                n318 = Number To Decimal String(number=w381) -> (decimal integer string=w388:string)  [unwired: 1 in]
                                n319 = Number To Decimal String(number=w382) -> (decimal integer string=w389:string)  [unwired: 1 in]
                                n320 = Number To Decimal String(number=0) -> (decimal integer string=w384:string)  [unwired: 1 in]
                                n321 = Number To Decimal String(number=0) -> (decimal integer string=w386:string)  [unwired: 1 in]
                                n322 = local read "Generated Sequence"() -> (w391:string[][])
                                n323 = Build Array("Go Straight", w384, w385, w386, w387, w388, w389) -> (w390:string[])
                                n324 = Build Array (concatenate)(w391, w390) -> (w392:string[][])
                                n325 = local write "Generated Sequence"(w392) -> ()
                                }
                                }
                                }
                                frame #1 {
                                n326 = stacked-sequence {
                                frame #0 {
                                n327 = local read "Generated Sequence"() -> (w400:string[][])
                                n328 = Build Array("Write  Pole", "P", "0", "0", "0", "0") -> (w401:string[])
                                n329 = Build Array (concatenate)(w400, w401) -> (w399:string[][])
                                n330 = local write "Generated Sequence"(w399) -> ()
                                }
                                frame #1 {
                                n331 = local read "X_axis(Inc)"() -> (w415:string)
                                n332 = local read "Y_axis(Inc)"() -> (w414:string)
                                n333 = local read "Z_axis(Inc)"() -> (w413:string)
                                n334 = case shown="\"Right\", Default" w415 {
                                tunnel: [0 1] -> w417
                                frame "Right", Default {
                                }
                                frame "Left" {
                                }
                                }
                                n335 = case shown="\"Back\", Default" w414 {
                                tunnel: [1 0] -> w418
                                frame "Back", Default {
                                }
                                frame "Front" {
                                }
                                }
                                n336 = case shown="\"Down\", Default" w413 {
                                tunnel: [0 1] -> w419
                                frame "Down", Default {
                                }
                                frame "Up" {
                                }
                                }
                                n337 = local read "Pole width N"() -> (w416:dbl)
                                n338 = Number To Decimal String(number=w416) -> (decimal integer string=w421:string)  [unwired: 1 in]
                                n339 = Number To Decimal String(number=w417) -> (decimal integer string=w423:string)  [unwired: 1 in]
                                n340 = Number To Decimal String(number=w418) -> (decimal integer string=w424:string)  [unwired: 1 in]
                                n341 = Number To Decimal String(number=w419) -> (decimal integer string=w425:string)  [unwired: 1 in]
                                n342 = local read "Generated Sequence"() -> (w412:string[][])
                                n343 = Number To Decimal String(number=0) -> (decimal integer string=w420:string)  [unwired: 1 in]
                                n344 = Number To Decimal String(number=0) -> (decimal integer string=w422:string)  [unwired: 1 in]
                                n345 = Build Array("Go Straight", w420, w421, w422, w423, w424, w425) -> (w426:string[])
                                n346 = Build Array (concatenate)(w412, w426) -> (w411:string[][])
                                n347 = local write "Generated Sequence"(w411) -> ()
                                }
                                }
                                }
                                }
                                }
                              }
                              frame #1 {
                                n348 = property on="Write_Menu" class="TabCtl (strict)"() -> ("Pages"=w434:refnum<vi>[])  [unwired: 2 in, 2 out]
                                n349 = Index Array(array=w434, index=3) -> (element=w435:refnum<vi>)
                                n350 = property on="Write_Menu" class="TabCtl (strict)"("Value"=T8."4.Save Script") -> ()  [unwired: 2 in, 2 out]
                                n351 = property class="Page"(reference=w435, "PageEnb"=T6."Page Enabled" ("Page Enabled State")) -> ()  [unwired: 1 in, 2 out]
                              }
                            }
                          }
                          frame "North", Default {
                            n352 = flat-sequence {
                              frame #0 {
                                n353 = local read "Pole width N"() -> (w440:dbl)
                                n354 = local read "Pole width S"() -> (w439:dbl)
                                n355 = local read "Strip Length"() -> (w442:dbl)
                                n356 = Add(x=w440, y=w439) -> (x+y=w438:dbl)
                                n357 = Divide(x=w442, y=w438) -> (x/y=w441:dbl)
                                n358 = for {
                                N: w441 -> [_]
                                n359 = flat-sequence {
                                frame #0 {
                                n360 = stacked-sequence {
                                frame #0 {
                                n361 = Build Array("Write  Pole", "P", "0", "0", "0", "0") -> (w444:string[])
                                n362 = local read "Generated Sequence"() -> (w445:string[][])
                                n363 = Build Array (concatenate)(w445, w444) -> (w443:string[][])
                                n364 = local write "Generated Sequence"(w443) -> ()
                                }
                                frame #1 {
                                n365 = case shown="\"Right\", Default" "X_axis(Inc)" {
                                tunnel: [0 1] -> w458
                                frame "Right", Default {
                                }
                                frame "Left" {
                                }
                                }
                                n366 = case shown="\"Back\", Default" "Y_axis(Inc)" {
                                tunnel: [1 0] -> w459
                                frame "Back", Default {
                                }
                                frame "Front" {
                                }
                                }
                                n367 = case shown="\"Down\", Default" "Z_axis(Inc)" {
                                tunnel: [0 1] -> w460
                                frame "Down", Default {
                                }
                                frame "Up" {
                                }
                                }
                                n368 = local read "Pole width N"() -> (w454:dbl)
                                n369 = Number To Decimal String(number=w454) -> (decimal integer string=w463:string)  [unwired: 1 in]
                                n370 = Number To Decimal String(number=w458) -> (decimal integer string=w465:string)  [unwired: 1 in]
                                n371 = Number To Decimal String(number=w459) -> (decimal integer string=w466:string)  [unwired: 1 in]
                                n372 = Number To Decimal String(number=w460) -> (decimal integer string=w467:string)  [unwired: 1 in]
                                n373 = Number To Decimal String(number=0) -> (decimal integer string=w462:string)  [unwired: 1 in]
                                n374 = Number To Decimal String(number=0) -> (decimal integer string=w464:string)  [unwired: 1 in]
                                n375 = local read "Generated Sequence"() -> (w469:string[][])
                                n376 = Build Array("Go Straight", w462, w463, w464, w465, w466, w467) -> (w468:string[])
                                n377 = Build Array (concatenate)(w469, w468) -> (w470:string[][])
                                n378 = local write "Generated Sequence"(w470) -> ()
                                }
                                }
                                }
                                frame #1 {
                                n379 = stacked-sequence {
                                frame #0 {
                                n380 = local read "Generated Sequence"() -> (w478:string[][])
                                n381 = Build Array("Write  Pole", "N", "0", "0", "0", "0") -> (w479:string[])
                                n382 = Build Array (concatenate)(w478, w479) -> (w477:string[][])
                                n383 = local write "Generated Sequence"(w477) -> ()
                                }
                                frame #1 {
                                n384 = local read "X_axis(Inc)"() -> (w493:string)
                                n385 = local read "Y_axis(Inc)"() -> (w492:string)
                                n386 = local read "Z_axis(Inc)"() -> (w491:string)
                                n387 = case shown="\"Right\", Default" w493 {
                                tunnel: [0 1] -> w495
                                frame "Right", Default {
                                }
                                frame "Left" {
                                }
                                }
                                n388 = case shown="\"Back\", Default" w492 {
                                tunnel: [1 0] -> w496
                                frame "Back", Default {
                                }
                                frame "Front" {
                                }
                                }
                                n389 = case shown="\"Down\", Default" w491 {
                                tunnel: [0 1] -> w497
                                frame "Down", Default {
                                }
                                frame "Up" {
                                }
                                }
                                n390 = local read "Pole width S"() -> (w494:dbl)
                                n391 = Number To Decimal String(number=w494) -> (decimal integer string=w499:string)  [unwired: 1 in]
                                n392 = Number To Decimal String(number=w495) -> (decimal integer string=w501:string)  [unwired: 1 in]
                                n393 = Number To Decimal String(number=w496) -> (decimal integer string=w502:string)  [unwired: 1 in]
                                n394 = Number To Decimal String(number=w497) -> (decimal integer string=w503:string)  [unwired: 1 in]
                                n395 = local read "Generated Sequence"() -> (w490:string[][])
                                n396 = Number To Decimal String(number=0) -> (decimal integer string=w498:string)  [unwired: 1 in]
                                n397 = Number To Decimal String(number=0) -> (decimal integer string=w500:string)  [unwired: 1 in]
                                n398 = Build Array("Go Straight", w498, w499, w500, w501, w502, w503) -> (w504:string[])
                                n399 = Build Array (concatenate)(w490, w504) -> (w489:string[][])
                                n400 = local write "Generated Sequence"(w489) -> ()
                                }
                                }
                                }
                                }
                                }
                              }
                              frame #1 {
                                n401 = property on="Write_Menu" class="TabCtl (strict)"() -> ("Pages"=w512:refnum<vi>[])  [unwired: 2 in, 2 out]
                                n402 = Index Array(array=w512, index=3) -> (element=w513:refnum<vi>)
                                n403 = property on="Write_Menu" class="TabCtl (strict)"("Value"=T8."4.Save Script") -> ()  [unwired: 2 in, 2 out]
                                n404 = property class="Page"(reference=w513, "PageEnb"=T6."Page Enabled" ("Page Enabled State")) -> ()  [unwired: 1 in, 2 out]
                              }
                            }
                          }
                        }
                      }
                    }
                  }
                }
              }
              frame "4.Save Script" {
                n405 = case shown="True" "Generate W4" {
                  frame False {
                  }
                  frame True {
                    n406 = flat-sequence {
                      frame #0 {
                        n407 = local read "Generated Sequence"() -> (w520:string[][])
                        n408 = Build Array("Home Position") -> (w519:string[])
                        n409 = Build Array (concatenate)(w520, w519) -> (w517:string[][])
                        n410 = local write "Generated Sequence"(w517) -> ()
                      }
                      frame #1 {
                        n411 = local read "Generated Sequence"() -> (w523:string[][])
                        n412 = Build Array("Sequence Stop") -> (w524:string[])
                        n413 = Build Array (concatenate)(w523, w524) -> (w522:string[][])
                        n414 = local write "Generated Sequence"(w522) -> ()
                      }
                      frame #2 {
                        n415 = local read "Generated Sequence"() -> (w526:string[][])
                        n416 = call-poly <vilib>:"Write To Spreadsheet File.vi"("2D data"=w526, "file path (dialog if empty)"="File Path_Write") -> ()  [unwired: 6 in, 1 out]
                      }
                      frame #3 {
                        n417 = One Button Dialog(message="New Script saved", button name ("OK")="OK") -> ()  [unwired: 1 out]
                      }
                    }
                  }
                }
              }
            }
          }
          frame "Read" {
            n418 = case shown="\"2.Sensors\"" "Read_Menu" {
              frame "1.Steps & Count", Default {
                n419 = case shown="True" "Generate R1" {
                  frame False {
                  }
                  frame True {
                    n420 = flat-sequence {
                      frame #0 {
                        n421 = case shown="\"Right\", Default" "X(R)" {
                          tunnel: [0 1] -> w543
                          frame "Right", Default {
                          }
                          frame "Left" {
                          }
                        }
                        n422 = case shown="\"Front\"" "Y(R)" {
                          tunnel: [1 0] -> w544
                          frame "Back", Default {
                          }
                          frame "Front" {
                          }
                        }
                        n423 = case shown="\"Down\", Default" "Z(R)" {
                          tunnel: [0 1] -> w545
                          frame "Down", Default {
                          }
                          frame "Up" {
                          }
                        }
                        n424 = local read "Xaxis"() -> (w537:dbl)
                        n425 = local read "Yaxis"() -> (w536:dbl)
                        n426 = local read "Zaxis"() -> (w535:dbl)
                        n427 = Format Into String(format string="%5.1f", w537) -> (resulting string=w550:string)  [unwired: 2 in, 1 out]
                        n428 = Format Into String(format string="%5.1f", w536) -> (resulting string=w552:string)  [unwired: 2 in, 1 out]
                        n429 = Format Into String(format string="%5.1f", w535) -> (resulting string=w551:string)  [unwired: 2 in, 1 out]
                        n430 = Number To Decimal String(number=w543) -> (decimal integer string=w546:string)  [unwired: 1 in]
                        n431 = Number To Decimal String(number=w544) -> (decimal integer string=w547:string)  [unwired: 1 in]
                        n432 = Number To Decimal String(number=w545) -> (decimal integer string=w548:string)  [unwired: 1 in]
                        n433 = local read "Generated Sequence"() -> (w539:string[][])
                        n434 = Build Array("Set Steps", w550, w552, w551, w546, w547, w548) -> (w549:string[])
                        n435 = Build Array (concatenate)(w539, w549) -> (w538:string[][])
                        n436 = local write "Generated Sequence"(w538) -> ()
                      }
                      frame #1 {
                        w568 = 0
                        n437 = local read "Xaxis"() -> (w571:dbl)
                        n438 = local read "Yaxis"() -> (w570:dbl)
                        n439 = local read "Zaxis"() -> (w569:dbl)
                        n440 = Equal?(x=w571, y=w568) -> (x = y?=w567:bool)
                        n441 = Equal?(x=w570, y=w568) -> (x = y?=w566:bool)
                        n442 = Equal?(x=w569, y=w568) -> (x = y?=w565:bool)
                        n443 = local read "Count"() -> (w564:dbl)
                        n444 = case shown="False" w567 {
                          frame False {
                            n445 = local read "Strip_Length"() -> (w580:dbl)
                            n446 = local read "Xaxis"() -> (w579:dbl)
                            n447 = Divide(x=w580, y=w579) -> (x/y=w578:dbl)
                            n448 = local write "Count"(w578) -> ()
                          }
                          frame True {
                          }
                        }
                        n449 = case shown="False" w566 {
                          frame False {
                            n450 = local read "Strip_Length"() -> (w577:dbl)
                            n451 = local read "Yaxis"() -> (w576:dbl)
                            n452 = Divide(x=w577, y=w576) -> (x/y=w575:dbl)
                            n453 = local write "Count"(w575) -> ()
                          }
                          frame True {
                          }
                        }
                        n454 = case shown="False" w565 {
                          frame False {
                            n455 = local read "Strip_Length"() -> (w574:dbl)
                            n456 = local read "Z axis"() -> (w573:dbl)
                            n457 = Divide(x=w574, y=w573) -> (x/y=w572:dbl)
                            n458 = local write "Count"(w572) -> ()
                          }
                          frame True {
                          }
                        }
                        n459 = Number To Decimal String(number=w564) -> (decimal integer string=w563:string)  [unwired: 1 in]
                        n460 = local read "Generated Sequence"() -> (w561:string[][])
                        n461 = Build Array("Set Count", w563) -> (w560:string[])
                        n462 = Build Array (concatenate)(w561, w560) -> (w559:string[][])
                        n463 = local write "Generated Sequence"(w559) -> ()
                      }
                      frame #2 {
                        n464 = property on="Read_Menu" class="TabCtl (strict)"() -> ("Pages"=w582:refnum<vi>[])  [unwired: 2 in, 2 out]
                        n465 = property on="Read_Menu" class="TabCtl (strict)"("Value"=T7."2.Sensors") -> ()  [unwired: 2 in, 2 out]
                        n466 = Index Array(array=w582, index=1) -> (element=w583:refnum<vi>)
                        n467 = property class="Page"(reference=w583, "PageEnb"=T6."Page Enabled" ("Page Enabled State")) -> ()  [unwired: 1 in, 2 out]
                      }
                    }
                  }
                }
              }
              frame "2.Sensors" {
                n468 = case shown="True" "Generate R2" {
                  frame False {
                  }
                  frame True {
                    n469 = flat-sequence {
                      frame #0 {
                        n470 = case shown="True" "ED32i" {
                          frame False {
                          }
                          frame True {
                            n471 = local read "Generated Sequence"() -> (w601:string[][])
                            n472 = Build Array("Read Sensors", "ED32i") -> (w602:string[])
                            n473 = Build Array (concatenate)(w601, w602) -> (w600:string[][])
                            n474 = local write "Generated Sequence"(w600) -> ()
                          }
                        }
                        n475 = case shown="True" "ED33" {
                          frame False {
                          }
                          frame True {
                            n476 = local read "Generated Sequence"() -> (w596:string[][])
                            n477 = Build Array("Read Sensors", "ED33") -> (w597:string[])
                            n478 = Build Array (concatenate)(w596, w597) -> (w595:string[][])
                            n479 = local write "Generated Sequence"(w595) -> ()
                          }
                        }
                        n480 = case shown="True" "KMT" {
                          frame False {
                          }
                          frame True {
                            n481 = local read "Generated Sequence"() -> (w591:string[][])
                            n482 = Build Array("Read Sensors", "ED33") -> (w592:string[])
                            n483 = Build Array (concatenate)(w591, w592) -> (w590:string[][])
                            n484 = local write "Generated Sequence"(w590) -> ()
                          }
                        }
                      }
                      frame #1 {
                        n485 = case shown="True" "Continuous" {
                          frame False {
                          }
                          frame True {
                            n486 = local read "X(R)"() -> (w614:string)
                            n487 = local read "Y(R)"() -> (w613:string)
                            n488 = local read "Z(R)"() -> (w612:string)
                            n489 = case shown="\"Right\", Default" w614 {
                              tunnel: [0 1] -> w619
                              frame "Right", Default {
                              }
                              frame "Left" {
                              }
                            }
                            n490 = case shown="\"Front\"" w613 {
                              tunnel: [1 0] -> w618
                              frame "Back", Default {
                              }
                              frame "Front" {
                              }
                            }
                            n491 = case shown="\"Down\", Default" w612 {
                              tunnel: [0 1] -> w617
                              frame "Down", Default {
                              }
                              frame "Up" {
                              }
                            }
                            n492 = local read "Xaxis"() -> (w609:dbl)
                            n493 = local read "Yaxis"() -> (w610:dbl)
                            n494 = local read "Zaxis"() -> (w611:dbl)
                            n495 = Format Into String(format string="%5.3f", w609) -> (resulting string=w620:string)  [unwired: 2 in, 1 out]
                            n496 = Format Into String(format string="%5.3f", w610) -> (resulting string=w621:string)  [unwired: 2 in, 1 out]
                            n497 = Format Into String(format string="%5.3f", w611) -> (resulting string=w622:string)  [unwired: 2 in, 1 out]
                            n498 = Number To Decimal String(number=w619) -> (decimal integer string=w623:string)  [unwired: 1 in]
                            n499 = Number To Decimal String(number=w618) -> (decimal integer string=w624:string)  [unwired: 1 in]
                            n500 = Number To Decimal String(number=w617) -> (decimal integer string=w625:string)  [unwired: 1 in]
                            n501 = local read "Generated Sequence"() -> (w608:string[][])
                            n502 = Build Array("Go Straight", w620, w621, w622, w623, w624, w625) -> (w615:string[])
                            n503 = Build Array (concatenate)(w608, w615) -> (w607:string[][])
                            n504 = local write "Generated Sequence"(w607) -> ()
                          }
                        }
                        n505 = case shown="True" "Move&Measure" {
                          frame False {
                          }
                          frame True {
                            n506 = local read "X(R)"() -> (w644:string)
                            n507 = local read "Y(R)"() -> (w643:string)
                            n508 = local read "Z(R)"() -> (w642:string)
                            n509 = case shown="\"Right\", Default" w644 {
                              tunnel: [0 1] -> w641
                              frame "Right", Default {
                              }
                              frame "Left" {
                              }
                            }
                            n510 = case shown="\"Front\"" w643 {
                              tunnel: [1 0] -> w640
                              frame "Back", Default {
                              }
                              frame "Front" {
                              }
                            }
                            n511 = case shown="\"Down\", Default" w642 {
                              tunnel: [0 1] -> w639
                              frame "Down", Default {
                              }
                              frame "Up" {
                              }
                            }
                            n512 = local read "Xaxis"() -> (w647:dbl)
                            n513 = local read "Yaxis"() -> (w646:dbl)
                            n514 = local read "Zaxis"() -> (w645:dbl)
                            n515 = Format Into String(format string="%5.3f", w647) -> (resulting string=w648:string)  [unwired: 2 in, 1 out]
                            n516 = Format Into String(format string="%5.3f", w646) -> (resulting string=w649:string)  [unwired: 2 in, 1 out]
                            n517 = Format Into String(format string="%5.3f", w645) -> (resulting string=w650:string)  [unwired: 2 in, 1 out]
                            n518 = Number To Decimal String(number=w641) -> (decimal integer string=w651:string)  [unwired: 1 in]
                            n519 = Number To Decimal String(number=w640) -> (decimal integer string=w652:string)  [unwired: 1 in]
                            n520 = Number To Decimal String(number=w639) -> (decimal integer string=w653:string)  [unwired: 1 in]
                            n521 = local read "Generated Sequence"() -> (w635:string[][])
                            n522 = Build Array("Move & Measure", w648, w649, w650, w651, w652, w653) -> (w637:string[])
                            n523 = Build Array (concatenate)(w635, w637) -> (w636:string[][])
                            n524 = local write "Generated Sequence"(w636) -> ()
                          }
                        }
                      }
                      frame #2 {
                        n525 = local read "Generated Sequence"() -> (w665:string[][])
                        n526 = Build Array("Clear SensorReadings") -> (w666:string[])
                        n527 = Build Array (concatenate)(w665, w666) -> (w664:string[][])
                        n528 = local write "Generated Sequence"(w664) -> ()
                      }
                      frame #3 {
                        n529 = property on="Read_Menu" class="TabCtl (strict)"() -> ("Pages"=w668:refnum<vi>[])  [unwired: 2 in, 2 out]
                        n530 = Index Array(array=w668, index=2) -> (element=w669:refnum<vi>)
                        n531 = property on="Read_Menu" class="TabCtl (strict)"("Value"=T7."3.Save Script") -> ()  [unwired: 2 in, 2 out]
                        n532 = property class="Page"(reference=w669, "PageEnb"=T6."Page Enabled" ("Page Enabled State")) -> ()  [unwired: 1 in, 2 out]
                      }
                    }
                  }
                }
              }
              frame "3.Save Script" {
                n533 = case shown="True" "Generate R4" {
                  frame False {
                  }
                  frame True {
                    n534 = flat-sequence {
                      frame #0 {
                        n535 = local read "Generated Sequence"() -> (w674:string[][])
                        n536 = Build Array("Sequence Stop") -> (w675:string[])
                        n537 = Build Array (concatenate)(w674, w675) -> (w673:string[][])
                        n538 = local write "Generated Sequence"(w673) -> ()
                      }
                      frame #1 {
                        n539 = local read "Generated Sequence"() -> (w678:string[][])
                        n540 = call-poly <vilib>:"Write To Spreadsheet File.vi"("2D data"=w678, "file path (dialog if empty)"="File Path_Read") -> ()  [unwired: 6 in, 1 out]
                      }
                      frame #2 {
                        n541 = One Button Dialog(message="New Script saved", button name ("OK")="OK") -> ()  [unwired: 1 out]
                      }
                    }
                  }
                }
              }
            }
          }
        }
        n542 = global write "Global_Not-Aus.vi" "Not-Aus"("Stop Program") -> ()
      }
    }
  }
